vi "纳清探头校准.vi"(5 "校准方式":u16, 6 "MB_Master输入":refnum<class "MB_Master.lvclass">, 7 "探头":T1(ring), 8 "错误输入（无错误）":errorcluster, 9 "标液三":cluster{"标准值":dbl, "检测值":dbl, "原始值":dbl}, 10 "标液二":cluster{"标准值":dbl, "检测值":dbl, "原始值":dbl}, 11 "标液一":cluster{"标准值":dbl, "检测值":dbl, "原始值":dbl}) -> (0 "错误输出":errorcluster)   [LabVIEW 2016, in "斯坦道多参数.lvlib"]
uses:
  <vilib>/Plasmionique/MB Master/MB_Master/MB_Master.lvclass
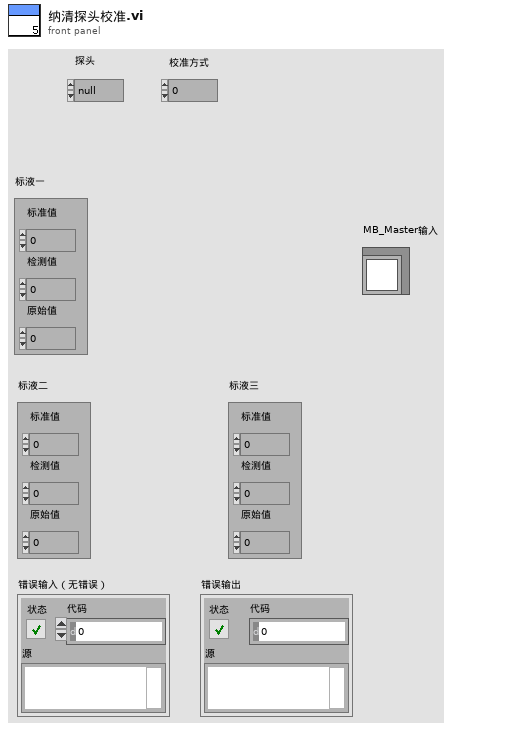
[diagram p1: front panel]
types:
  T1 = enum16{"null", "pH", "DO", "浊度", "电导率", "叶绿素a", "藻密度"}
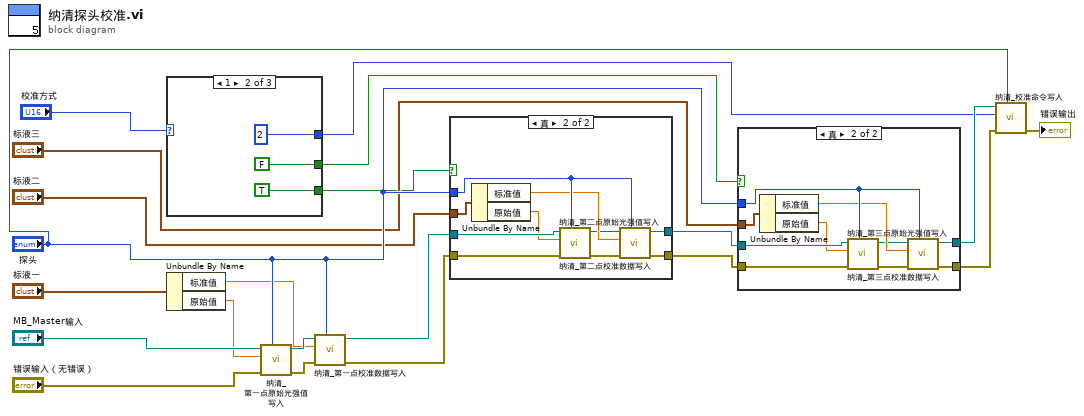
[diagram p0: block diagram]
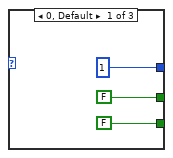
[diagram p4: hidden frame]
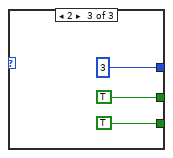
[diagram p5: hidden frame]
diagram:
  n1 = case shown="1" "校准方式" {
    tunnel: [u16 1 ("数值") u16 2 ("数值") u16 3 ("数值")] -> w5
    tunnel: [FALSE TRUE TRUE] -> w4
    tunnel: [FALSE FALSE TRUE] -> w3
    frame 0, Default {
    }
    frame 1 {
    }
    frame 2 {
    }
  }
  n2 = Unbundle By Name("标液一") -> ("标准值"=w7:dbl, "原始值"=w8:dbl)
  n3 = call "纳清_第一点原始光强值写入.vi"("探头"="探头", "error in (no error)"="错误输入（无错误）", "数值"=w8, "MB session in"="MB_Master输入") -> ("error out"=w19:errorcluster, "MB session out"=w20:refnum<class "MB_Master.lvclass">)  [unwired: 6 in]
  n4 = call "纳清_第一点校准数据写入.vi"("探头"="探头", "error in (no error)"=w19, "数值"=w7, "MB session in"=w20) -> ("error out"=w17:errorcluster, "MB session out"=w11:refnum<class "MB_Master.lvclass">)  [unwired: 6 in]
  n5 = case shown="真" w4 {
    tunnel: "标液二" -> [_ w42]
    tunnel: w17 -> [w31 w41]
    tunnel: [w31 w40] -> w16
    tunnel: [w32 w39] -> w12
    tunnel: w11 -> [w32 w38]
    tunnel: "探头" -> [_ w37]
    frame False {
    }
    frame True {
      n6 = Unbundle By Name(w42) -> ("标准值"=w35:dbl, "原始值"=w36:dbl)
      n7 = call "纳清_第二点原始光强值写入.vi"("探头"=w37, "error in (no error)"=w41, "数值"=w36, "MB session in"=w38) -> ("error out"=w34:errorcluster, "MB session out"=w33:refnum<class "MB_Master.lvclass">)  [unwired: 6 in]
      n8 = call "纳清_第二点校准数据写入.vi"("探头"=w37, "error in (no error)"=w34, "数值"=w35, "MB session in"=w33) -> ("error out"=w40:errorcluster, "MB session out"=w39:refnum<class "MB_Master.lvclass">)  [unwired: 6 in]
    }
  }
  n9 = case shown="真" w3 {
    tunnel: w16 -> [w43 w54]
    tunnel: [w43 w53] -> w15
    tunnel: [w44 w52] -> w13
    tunnel: w12 -> [w44 w51]
    tunnel: "探头" -> [_ w50]
    tunnel: "标液三" -> [_ w49]
    frame False {
    }
    frame True {
      n10 = Unbundle By Name(w49) -> ("标准值"=w47:dbl, "原始值"=w48:dbl)
      n11 = call "纳清_第三点原始光强值写入.vi"("探头"=w50, "error in (no error)"=w54, "数值"=w48, "MB session in"=w51) -> ("error out"=w46:errorcluster, "MB session out"=w45:refnum<class "MB_Master.lvclass">)  [unwired: 6 in]
      n12 = call "纳清_第三点校准数据写入.vi"("探头"=w50, "error in (no error)"=w46, "数值"=w47, "MB session in"=w45) -> ("error out"=w53:errorcluster, "MB session out"=w52:refnum<class "MB_Master.lvclass">)  [unwired: 6 in]
    }
  }
  n13 = call "纳清_校准命令写入.vi"("探头"="探头", "error in (no error)"=w15, "数值"=w5, "MB session in"=w13) -> ("error out"=→"错误输出":errorcluster)  [unwired: 6 in, 1 out]
